vi "Cents2DollarString.vi"(11 "Cents In":dbl) -> (0 "Dollar Numeric Out":dbl, 3 "Dollar String Out":string)   [LabVIEW 2019]
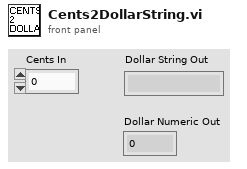
[diagram p1: front panel]
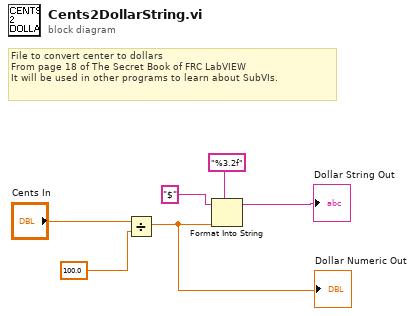
[diagram p0: block diagram]
diagram:
  # "File to convert center to dollars\nFrom page 18 of The Secret Book of FRC LabVIEW\nIt will be used in other programs to learn about SubVIs."
  n1 = Divide(x="Cents In", y=100.0 ("x/y")) -> (x/y=w1:dbl)
  "Dollar Numeric Out" <- w1
  n2 = Format Into String(format string="%3.2f", initial string="$", w1) -> (resulting string=→"Dollar String Out":string)  [unwired: 1 in, 1 out]
